vi "三菱PLC通讯.vi"(4 "等待时间（毫秒）":u32=50, 6 "stop bits (10: 1 bit)":u16(ring)=10 caption="停止位（10: 1位）" items=["1.0"=10, "1.5"=15, "2.0"=20], 8 "parity (0:none)":enum16{"None", "Odd", "Even", "Mark", "Space"}(ring)=enum."Even" caption="奇偶（0:无）", 9 "data bits (8)":u16=7 caption="数据比特(8)" min=5 max=8 step=1, 10 "baud rate (9600)":u32=9600 caption="波特率(9600)", 11 "VISA resource name":refnum<visa-resource-name> caption="VISA资源名称") -> ()   [LabVIEW 2014]
uses:
  <vilib>/Instr/_visa.llb/VISA Configure Serial Port (Instr).vi
panel:
  out "求和校验码":string
  out "子字符串":string
  out "字符串":string
  out "写数据":string
  out "读数据":string
  out "读取缓冲区":string
  in  "打开串口":bool
  out "read buffer":string
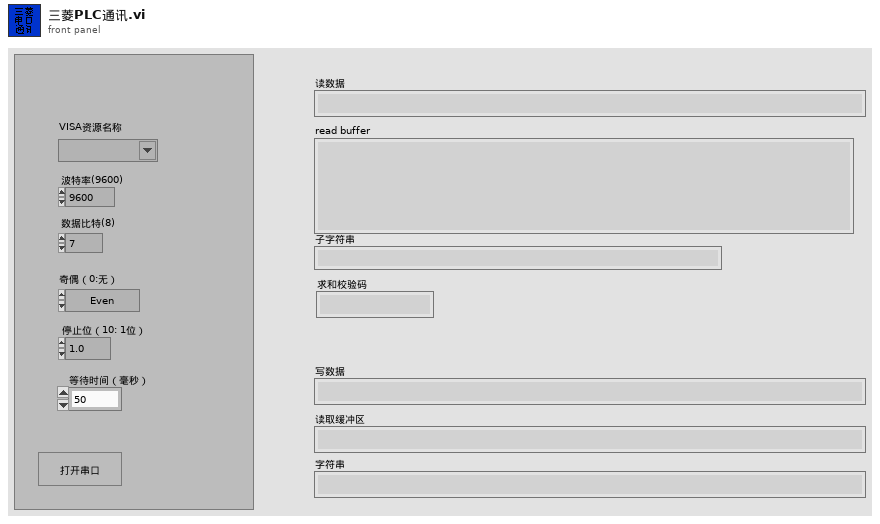
[diagram p1: front panel]
types:
  T1 = enum16{"等待", "打开串口", "关闭串口", "通讯失败", "读数据", "写数据"}
  T2 = cluster{"通讯串口":refnum<visa-resource-name>, "波特率":u32, "数据比特":u16, "奇偶校验":enum16{"None", "Odd", "Even", "Mark", "Space"}, "停止位":u16, "等待延时(ms)":u32}
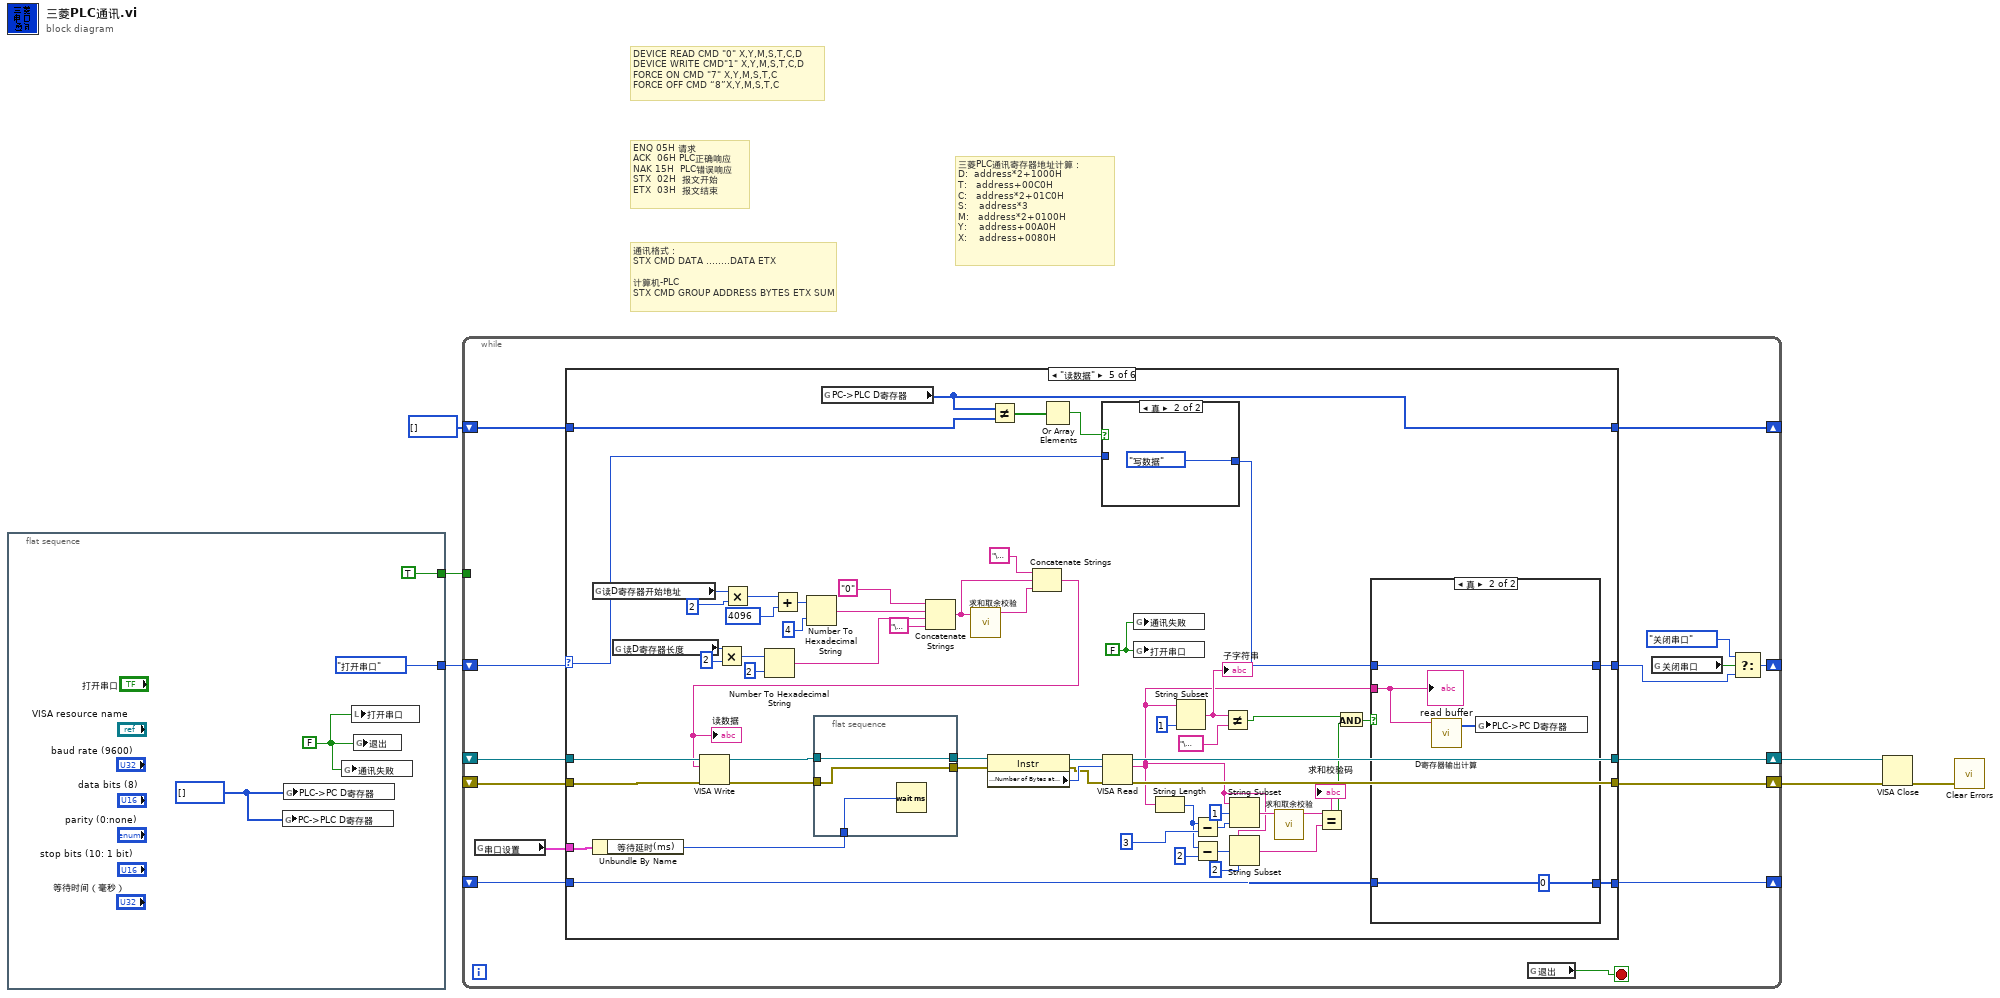
[diagram p0: block diagram]
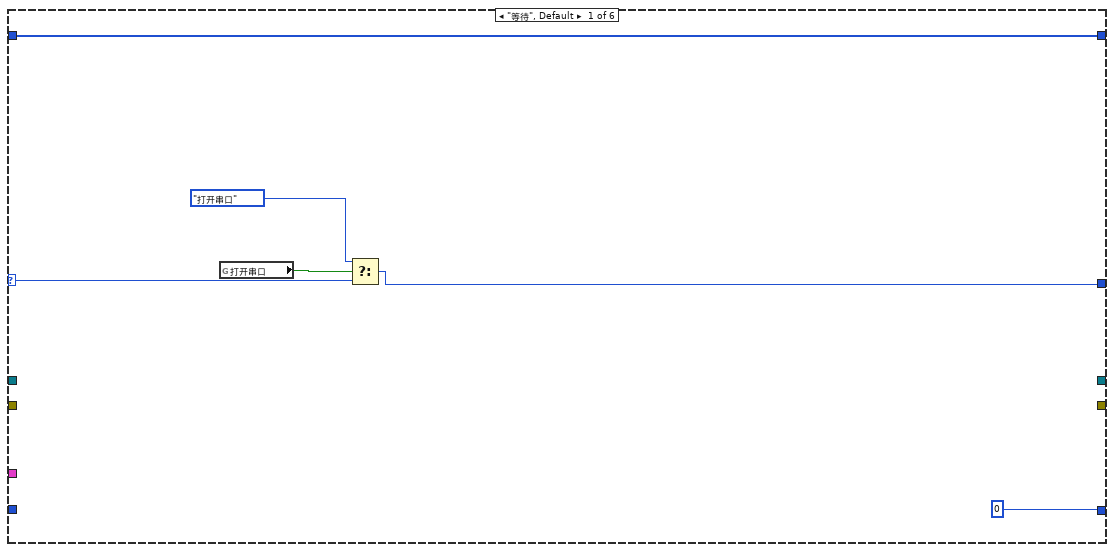
[diagram p2: hidden frame]
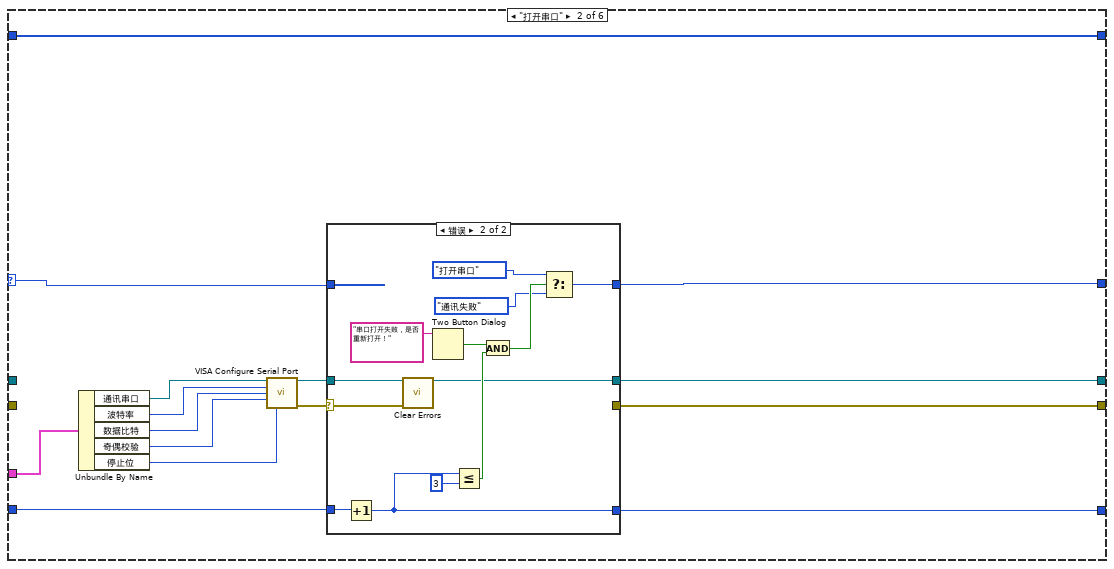
[diagram p3: hidden frame]
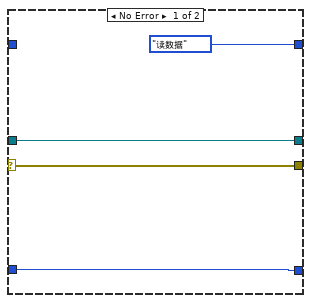
[diagram p4: hidden frame]
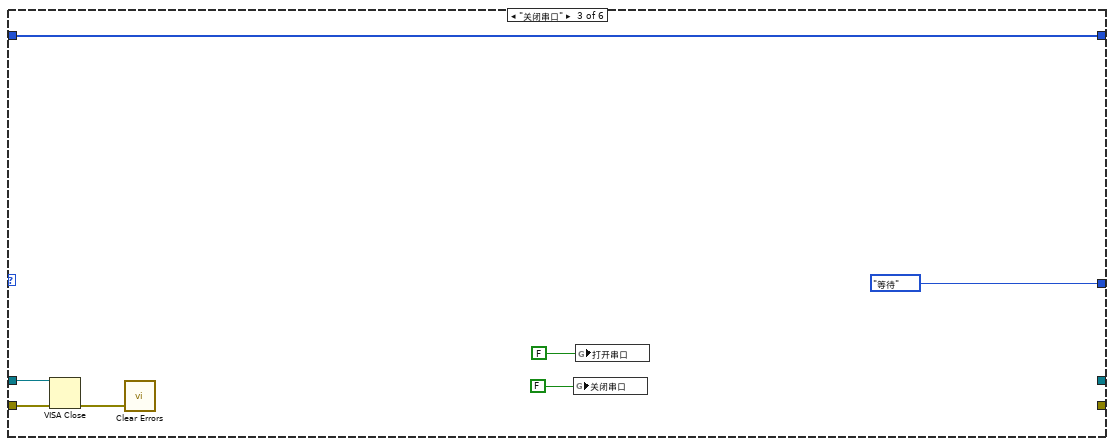
[diagram p5: hidden frame]
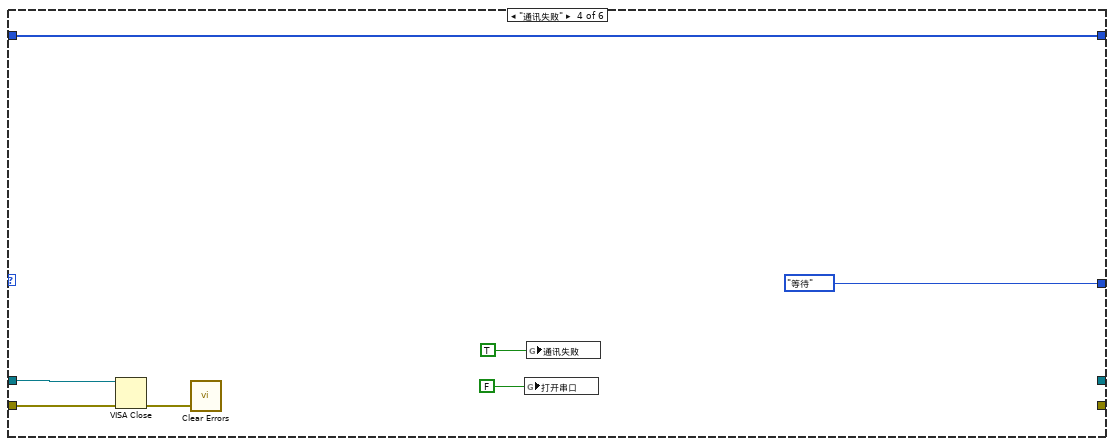
[diagram p6: hidden frame]
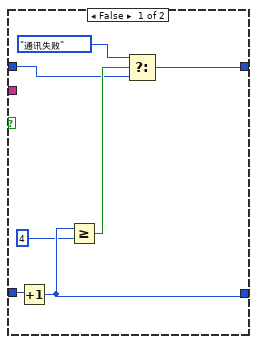
[diagram p8: hidden frame]
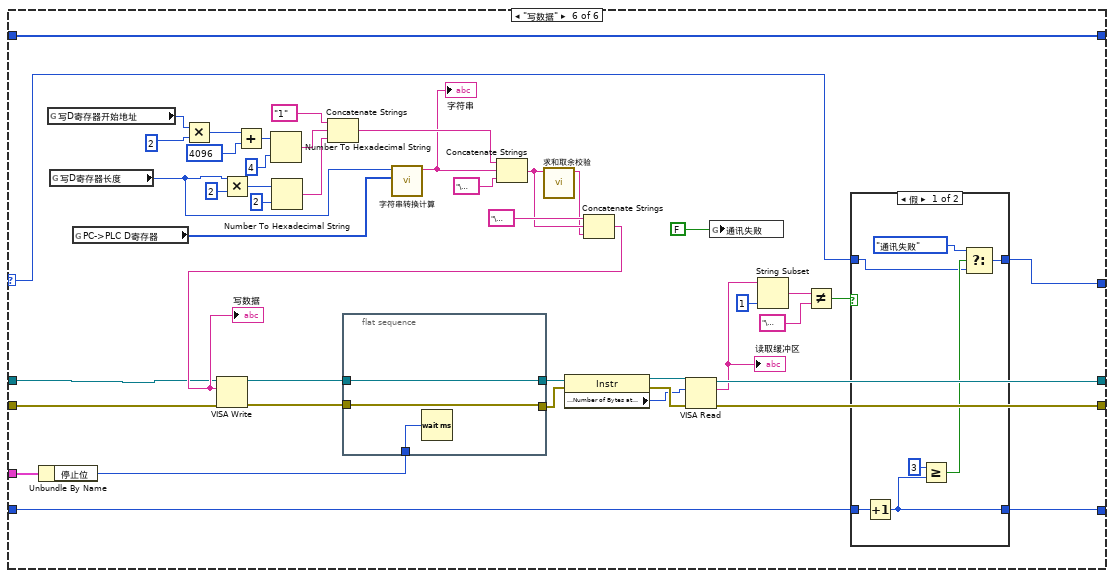
[diagram p9: hidden frame]
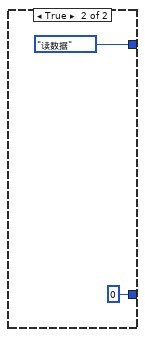
[diagram p10: hidden frame]
diagram:
  # "三菱PLC通讯寄存器地址计算：\nD:  address*2+1000H\nT:   address+00C0H\nC:   address*2+01C0H\nS:    address*3\nM:   address*2+0100H\nY:    address+00A0H\nX:    address+0080H"
  # "通讯格式：\nSTX CMD DATA ........DATA ETX\n\n计算机-PLC\nSTX CMD GROUP ADDRESS BYTES ETX SUM"
  # "ENQ 05H 请求\nACK  06H PLC正确响应\nNAK 15H  PLC错误响应\nSTX  02H  报文开始\nETX  03H  报文结束"
  # "DEVICE READ CMD \"0\" X,Y,M,S,T,C,D\nDEVICE WRITE CMD\"1\" X,Y,M,S,T,C,D\nFORCE ON CMD \"7\" X,Y,M,S,T,C\nFORCE OFF CMD “8”X,Y,M,S,T,C"
  n1 = flat-sequence {
    tunnel: [TRUE] -> w6
    tunnel: [T1."打开串口" ("通讯")] -> w5
    frame #0 {
      w8 = i16[] [] ("PC->PLC D寄存器")
      w7 = FALSE ("退出")
      n2 = global write "三菱全局变量.vi" "PC->PLC D寄存器"(w8) -> ()
      n3 = global write "三菱全局变量.vi" "PLC->PC D寄存器"(w8) -> ()
      n4 = global write "三菱全局变量.vi" "通讯失败"(w7) -> ()
      n5 = local write "打开串口"(w7) -> ()
      n6 = global write "三菱全局变量.vi" "退出"(w7) -> ()
    }
  }
  n7 = while {
    tunnel: w6 -> [_]
    shift-right: [w13] -> _
    shift-left: w5 -> [w25]
    shift-right: [w24] -> w3
    shift-left: _ -> [w22]
    shift-right: [w23] -> w2
    shift-left: _ -> [w21]
    shift-right: [w19] -> _
    shift-left: _ -> [w20]
    shift-right: [w16] -> _
    shift-left: i16[] [] ("PC->PLC D寄存器") -> [w17]
    stop <- w18 stop-if-true
    n8 = global read "三菱全局变量.vi" "串口设置"() -> (w11:T2)
    n9 = case shown="\"读数据\"" w25 {
      selector: w25 -> [w30 w45 _ _ w97 w161]
      tunnel: [w29 w44 T1."等待" ("通讯") T1."等待" ("通讯") w104 w160] -> w12
      tunnel: [_ w42 _ _ w108 w168] -> w24
      tunnel: [_ w41 _ _ w107 w167] -> w23
      tunnel: w22 -> [_ _ w68 w76 w118 w152]
      tunnel: w21 -> [_ _ w67 w75 w117 w151]
      tunnel: w20 -> [_ w40 _ _ w102 w159]
      tunnel: [0 w39 _ _ w103 w158] -> w19
      tunnel: w17 -> [w26 w38 w64 w71 w100 w157]
      tunnel: [w26 w38 w64 w71 w101 w157] -> w16
      tunnel: w11 -> [_ w37 _ _ w93 w155]
      frame "等待", Default {
        n10 = global read "三菱全局变量.vi" "打开串口"() -> (w31:bool)
        n11 = Select(t=T1."打开串口" ("通讯"), s=w31, f=w30) -> (s? t:f=w29:T1)
      }
      frame "打开串口" {
        n12 = Unbundle By Name(w37) -> ("通讯串口"=w36:refnum<visa-resource-name>, "波特率"=w35:u32, "数据比特"=w34:u16, "奇偶校验"=w33:enum16{"None", "Odd", "Even", "Mark", "Space"}, "停止位"=w32:u16)
        n13 = call-poly "VISA Configure Serial Port"("VISA resource name"=w36, "baud rate (9600)"=w35, "data bits (8)"=w34, "parity (0:none)"=w33, "stop bits (10: 1 bit)"=w32) -> ("VISA resource name out"=w43:refnum<visa-resource-name>, "error out"=w46:errorcluster)  [unwired: 9 in]
        n14 = case shown="错误" w46 {
          selector: w46 -> [w49 w51]
          tunnel: w45 -> [_ _]
          tunnel: [T1."读数据" ("通讯") w53] -> w44
          tunnel: w43 -> [w50 w52]
          tunnel: [w50 w52] -> w42
          tunnel: [w49 _] -> w41
          tunnel: w40 -> [w47 w62]
          tunnel: [w47 w60] -> w39
          frame No Error {
          }
          frame Error {
            n15 = Increment(x=w62) -> (x+1=w60:i32)
            n16 = call <vilib>:"Clear Errors.vi"("error in (no error)"=w51) -> ()  [unwired: 5 in, 2 out]
            n17 = Two Button Dialog(message="串口打开失败，是否重新打开！" ("消息")) -> (T button?=w57:bool)  [unwired: 2 in]
            n18 = Less Or Equal?(x=w60, y=3) -> (x <= y?=w58:bool)
            n19 = And(x=w57, y=w58) -> (x .and. y?=w56:bool)
            n20 = Select(t=T1."打开串口" ("通讯"), s=w56, f=T1."通讯失败" ("通讯")) -> (s? t:f=w53:T1)
          }
        }
      }
      frame "关闭串口" {
        n21 = VISA Close(VISA resource name=w68, error in (no error)=w67) -> (error out=w69:errorcluster)
        n22 = call <vilib>:"Clear Errors.vi"("error in (no error)"=w69) -> ()  [unwired: 5 in, 2 out]
        n23 = global write "三菱全局变量.vi" "关闭串口"(FALSE ("关闭串口")) -> ()
        n24 = global write "三菱全局变量.vi" "打开串口"(FALSE ("打开串口")) -> ()
      }
      frame "通讯失败" {
        n25 = VISA Close(VISA resource name=w76, error in (no error)=w75) -> (error out=w74:errorcluster)
        n26 = call <vilib>:"Clear Errors.vi"("error in (no error)"=w74) -> ()  [unwired: 5 in, 2 out]
        n27 = global write "三菱全局变量.vi" "打开串口"(FALSE ("打开串口")) -> ()
        n28 = global write "三菱全局变量.vi" "通讯失败"(TRUE ("打开串口")) -> ()
      }
      frame "读数据" {
        w91 = FALSE ("打开串口")
        n29 = global read "三菱全局变量.vi" "读D寄存器开始地址"() -> (w134:u16)
        n30 = Unbundle By Name(w93) -> ("等待延时(ms)"=w92:u32)
        n31 = global read "三菱全局变量.vi" "读D寄存器长度"() -> (w128:u16)
        n32 = Multiply(x=w128, y=u16 2) -> (x*y=w126:u16)
        n33 = Multiply(x=w134, y=u16 2) -> (x*y=w132:u16)
        n34 = Number To Hexadecimal String(1:i16 2 ("宽度(-)"), 2:w126) -> (0:w123:string)
        n35 = Add(x=w132, y=u16 4096) -> (x+y=w130:u16)
        n36 = Number To Hexadecimal String(1:i16 4 ("宽度(-)"), 2:w130) -> (0:w124:string)
        n37 = flat-sequence {
          tunnel: w112 -> [w150]
          tunnel: w111 -> [w149]
          tunnel: [w150] -> w110
          tunnel: [w149] -> w109
          tunnel: w92 -> [w148]
          frame #0 {
            n38 = Wait (ms)(milliseconds to wait=w148) -> ()  [unwired: 1 out]
          }
        }
        n39 = global read "三菱全局变量.vi" "PC->PLC D寄存器"() -> (w101:i16[])
        n40 = Concatenate Strings("0" ("字符串"), w124, w123, "\u0003" ("字符串")) -> (w120:string)
        n41 = call "求和取余校验.vi"("字符串"=w120) -> ("求和校验码"=w119:string)  [unwired: 10 in]
        n42 = property class="Instr"(reference=w110, error in=w109) -> (reference out=w115:refnum<visa-resource-name>, error out=w113:errorcluster, "Serial Settings:Number of Bytes at Serial Port"=w114:u32)
        n43 = Not Equal?(x=w101, y=w100) -> (x != y?=w99:bool[])
        n44 = Concatenate Strings("\u0002" ("字符串"), w120, w119) -> (w116:string)
        "读数据" <- w116
        n45 = VISA Write(VISA resource name=w118, write buffer=w116, error in (no error)=w117) -> (VISA resource name out=w112:refnum<visa-resource-name>, error out=w111:errorcluster)  [unwired: 1 out]
        n46 = Or Array Elements(Boolean array=w99) -> (logical OR=w98:bool)
        n47 = case shown="真" w98 {
          tunnel: w97 -> [w135 _]
          tunnel: [w135 T1."写数据" ("通讯")] -> w96
          frame False {
          }
          frame True {
          }
        }
        n48 = VISA Read(VISA resource name=w115, byte count=w114, error in (no error)=w113) -> (VISA resource name out=w108:refnum<visa-resource-name>, read buffer=w78:string, error out=w107:errorcluster)  [unwired: 1 out]
        n49 = global write "三菱全局变量.vi" "通讯失败"(w91) -> ()
        n50 = global write "三菱全局变量.vi" "打开串口"(w91) -> ()
        n51 = String Length(string=w78) -> (length=w77:i32)
        n52 = String Subset(string=w78, length (rest)=1 ("长度（剩余）")) -> (substring=w94:string)  [unwired: 1 in]
        "子字符串" <- w94
        n53 = Subtract(x=w77, y=3) -> (x-y=w89:i32)
        n54 = Subtract(x=w77, y=2) -> (x-y=w85:i32)
        n55 = Not Equal?(x=w94, y="\u0015" ("字符串")) -> (x != y?=w81:bool)
        n56 = String Subset(string=w78, offset (0)=1 ("偏移量(0)"), length (rest)=w89) -> (substring=w88:string)
        n57 = String Subset(string=w78, offset (0)=w85, length (rest)=2 ("长度（剩余）")) -> (substring=w82:string)
        n58 = call "求和取余校验.vi"("字符串"=w88) -> ("求和校验码"=w83:string)  [unwired: 10 in]
        "求和校验码" <- w83
        n59 = Equal?(x=w83, y=w82) -> (x = y?=w79:bool)
        n60 = And(x=w81, y=w79) -> (x .and. y?=w80:bool)
        n61 = case shown="真" w80 {
          tunnel: w96 -> [w138 w147]
          tunnel: [w142 w147] -> w104
          tunnel: [w141 0] -> w103
          tunnel: w102 -> [w143 _]
          tunnel: w78 -> [_ w145]
          frame False {
            n62 = Increment(x=w143) -> (x+1=w141:i32)
            n63 = Greater Or Equal?(x=w141, y=4) -> (x >= y?=w139:bool)
            n64 = Select(t=T1."通讯失败" ("通讯"), s=w139, f=w138) -> (s? t:f=w142:T1)
          }
          frame True {
            n65 = call "D寄存器输出计算.vi"("字符串"=w145) -> ("输出"=w144:u16[])  [unwired: 10 in]
            n66 = global write "三菱全局变量.vi" "PLC->PC D寄存器"(w144) -> ()
            "read buffer" <- w145
          }
        }
      }
      frame "写数据" {
        n67 = Unbundle By Name(w155) -> ("停止位"=w154:u16)
        n68 = global read "三菱全局变量.vi" "写D寄存器开始地址"() -> (w190:u16)
        n69 = global read "三菱全局变量.vi" "写D寄存器长度"() -> (w184:u16)
        n70 = global read "三菱全局变量.vi" "PC->PLC D寄存器"() -> (w183:i16[])
        n71 = Multiply(x=w190, y=u16 2) -> (x*y=w194:u16)
        n72 = Multiply(x=w184, y=u16 2) -> (x*y=w186:u16)
        n73 = Add(x=w194, y=u16 4096) -> (x+y=w192:u16)
        n74 = Number To Hexadecimal String(1:i16 4 ("宽度(-)"), 2:w192) -> (0:w188:string)
        n75 = Number To Hexadecimal String(1:i16 2 ("宽度(-)"), 2:w186) -> (0:w185:string)
        n76 = Concatenate Strings("1" ("字符串"), w188, w185) -> (w182:string)
        n77 = flat-sequence {
          tunnel: w175 -> [w206]
          tunnel: w174 -> [w205]
          tunnel: w154 -> [w207]
          tunnel: [w206] -> w173
          tunnel: [w205] -> w172
          frame #0 {
            n78 = Wait (ms)(milliseconds to wait=w207) -> ()  [unwired: 1 out]
          }
        }
        n79 = call "字符串转换计算.vi"("PC->PLC D寄存器"=w183, "读D寄存器长度"=w184) -> ("字符串"=w181:string)  [unwired: 9 in]
        "字符串" <- w181
        n80 = Concatenate Strings(w182, w181, "\u0003" ("字符串")) -> (w178:string)
        n81 = call "求和取余校验.vi"("字符串"=w178) -> ("求和校验码"=w177:string)  [unwired: 10 in]
        n82 = property class="Instr"(reference=w173, error in=w172) -> (reference out=w171:refnum<visa-resource-name>, error out=w170:errorcluster, "Serial Settings:Number of Bytes at Serial Port"=w169:u32)
        n83 = Concatenate Strings("\u0002" ("字符串"), w178, w177) -> (w176:string)
        "写数据" <- w176
        n84 = VISA Write(VISA resource name=w152, write buffer=w176, error in (no error)=w151) -> (VISA resource name out=w175:refnum<visa-resource-name>, error out=w174:errorcluster)  [unwired: 1 out]
        n85 = VISA Read(VISA resource name=w171, byte count=w169, error in (no error)=w170) -> (VISA resource name out=w168:refnum<visa-resource-name>, read buffer=w163:string, error out=w167:errorcluster)  [unwired: 1 out]
        "读取缓冲区" <- w163
        n86 = global write "三菱全局变量.vi" "通讯失败"(FALSE ("通讯失败")) -> ()
        n87 = String Subset(string=w163, length (rest)=1 ("长度（剩余）")) -> (substring=w164:string)  [unwired: 1 in]
        n88 = Not Equal?(x=w164, y="\u0015" ("字符串")) -> (x != y?=w162:bool)
        n89 = case shown="假" w162 {
          tunnel: w161 -> [w197 _]
          tunnel: [w199 T1."读数据" ("通讯")] -> w160
          tunnel: w159 -> [w202 _]
          tunnel: [w201 0] -> w158
          frame False {
            n90 = Increment(x=w202) -> (x+1=w201:i32)
            n91 = Greater Or Equal?(x=3, y=w201) -> (x >= y?=w198:bool)
            n92 = Select(t=T1."通讯失败" ("通讯"), s=w198, f=w197) -> (s? t:f=w199:T1)
          }
          frame True {
          }
        }
      }
    }
    n93 = global read "三菱全局变量.vi" "退出"() -> (w18:bool)
    n94 = global read "三菱全局变量.vi" "关闭串口"() -> (w15:bool)
    n95 = Select(t=T1."关闭串口" ("通讯"), s=w15, f=w12) -> (s? t:f=w13:T1)
  }
  n96 = VISA Close(VISA resource name=w3, error in (no error)=w2) -> (error out=w4:errorcluster)
  n97 = call <vilib>:"Clear Errors.vi"("error in (no error)"=w4) -> ()  [unwired: 5 in, 2 out]
